vi "ScanDelayGetDelayWaveform.vi"(8 "error in (no error)":errorcluster, 9 "wait":u32=10, 11 "VISA resource name in":refnum<visa-resource-name>) -> (0 "error out":errorcluster, 2 "values":i16[](array[numeric]), 3 "VISA resource name out":refnum<visa-resource-name>)   [LabVIEW 2018]
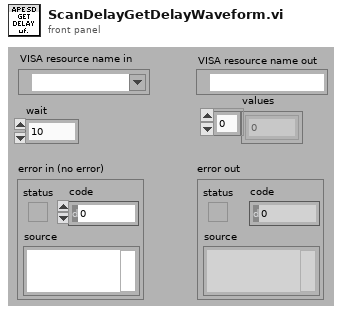
[diagram p1: front panel]
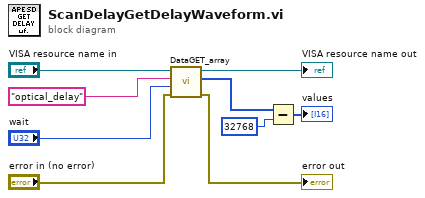
[diagram p0: block diagram]
diagram:
  n1 = call "DataGET_array.vi"("error in (no error)"="error in (no error)", "Wait"="wait", "parameter"="optical_delay", "VISA resource name"="VISA resource name in") -> ("error out"=→"error out":errorcluster, "PSD Waveform"=w3:u16[], "VISA resource name out"=→"VISA resource name out":refnum<visa-resource-name>)  [unwired: 4 in, 1 out]
  n2 = Subtract(x=w3, y=32768) -> (x-y=→"values":i32[])
